vi "WPI_ADI_IMU_RolloverFix.vi"(9 "Previous":T1, 10 "Current":T1) -> (2 "Output":T1)   [LabVIEW 2015]
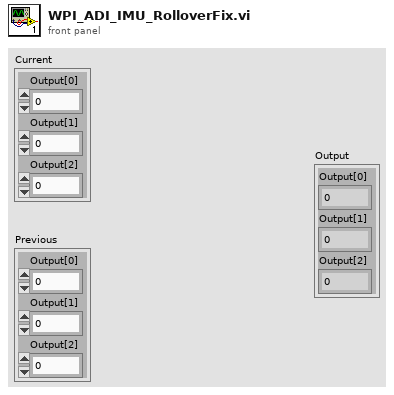
[diagram p1: front panel]
types:
  T1 = cluster{"Output[0]":dbl, "Output[1]":dbl, "Output[2]":dbl}
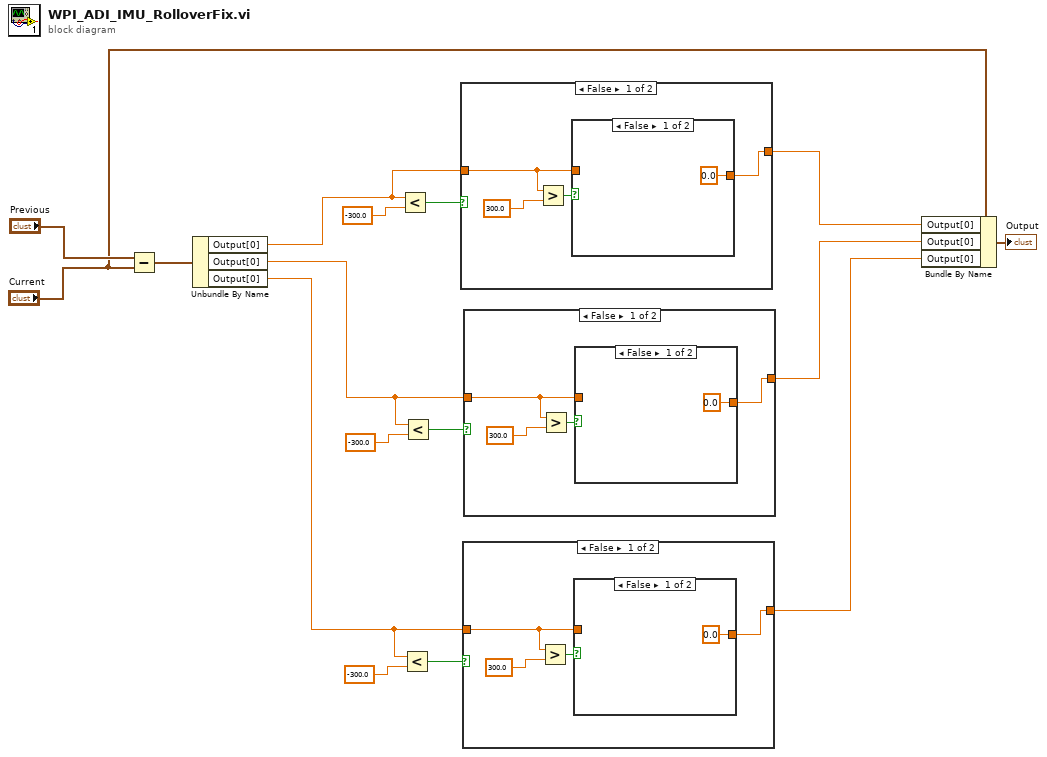
[diagram p0: block diagram]
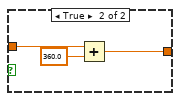
[diagram p2: hidden frame]
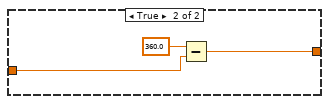
[diagram p3: hidden frame]
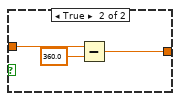
[diagram p4: hidden frame]
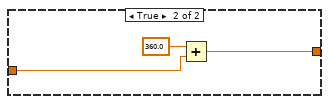
[diagram p5: hidden frame]
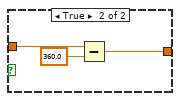
[diagram p6: hidden frame]
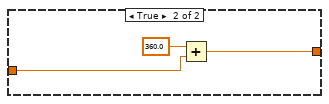
[diagram p7: hidden frame]
diagram:
  n1 = Subtract(x="Previous", y="Current") -> (x-y=w16:T1)
  n2 = Unbundle By Name(w16) -> ("Output[0]"=w13:dbl, "Output[0]"=w10:dbl, "Output[0]"=w7:dbl)
  n3 = Less?(x=w13, y=-300.0) -> (x < y?=w14:bool)
  n4 = Less?(x=w7, y=-300.0) -> (x < y?=w8:bool)
  n5 = Less?(x=w10, y=-300.0) -> (x < y?=w11:bool)
  n6 = case shown="False" w14 {
    tunnel: w13 -> [w18 w26]
    tunnel: [w17 w25] -> w6
    frame False {
      n7 = Greater?(x=w18, y=300.0) -> (0:w19:bool)
      n8 = case shown="False" w19 {
        tunnel: w18 -> [_ w24]
        tunnel: [0.0 w22] -> w17
        frame False {
        }
        frame True {
          n9 = Subtract(x=w24, y=360.0) -> (x-y=w22:dbl)
        }
      }
    }
    frame True {
      n10 = Add(x=360.0, y=w26) -> (x+y=w25:dbl)
    }
  }
  n11 = case shown="False" w8 {
    tunnel: w7 -> [w29 w37]
    tunnel: [w28 w36] -> w4
    frame False {
      n12 = Greater?(x=w29, y=300.0) -> (0:w30:bool)
      n13 = case shown="False" w30 {
        tunnel: w29 -> [_ w35]
        tunnel: [0.0 w33] -> w28
        frame False {
        }
        frame True {
          n14 = Add(x=w35, y=360.0) -> (x+y=w33:dbl)
        }
      }
    }
    frame True {
      n15 = Subtract(x=360.0, y=w37) -> (x-y=w36:dbl)
    }
  }
  n16 = case shown="False" w11 {
    tunnel: w10 -> [w40 w48]
    tunnel: [w39 w47] -> w5
    frame False {
      n17 = Greater?(x=w40, y=300.0) -> (0:w41:bool)
      n18 = case shown="False" w41 {
        tunnel: w40 -> [_ w46]
        tunnel: [0.0 w44] -> w39
        frame False {
        }
        frame True {
          n19 = Subtract(x=w46, y=360.0) -> (x-y=w44:dbl)
        }
      }
    }
    frame True {
      n20 = Add(x=360.0, y=w48) -> (x+y=w47:dbl)
    }
  }
  n21 = Bundle By Name(cluster="Current", "Output[0]"=w6, "Output[0]"=w5, "Output[0]"=w4) -> (→"Output":T1)
